vi "dump_photon_stream.vi"(5 "acq_mode":T1=2 items=["T2"=2, "T3"=3], 7 "sync":u64[](array[numeric]), 8 "error in (no error)":errorcluster, 9 "channels":u8[](array[numeric]), 10 "photon_records":u64[](array[numeric]), 11 "data_logger in":refnum<class "data_logger.lvclass">) -> (0 "error out":errorcluster, 3 "data_logger out":refnum<class "data_logger.lvclass">)   [LabVIEW 2015, in "data_logger.lvclass"]
uses:
  data_logger.lvclass
  lvoop_dll-master/picoquant_Tmodes.ctl
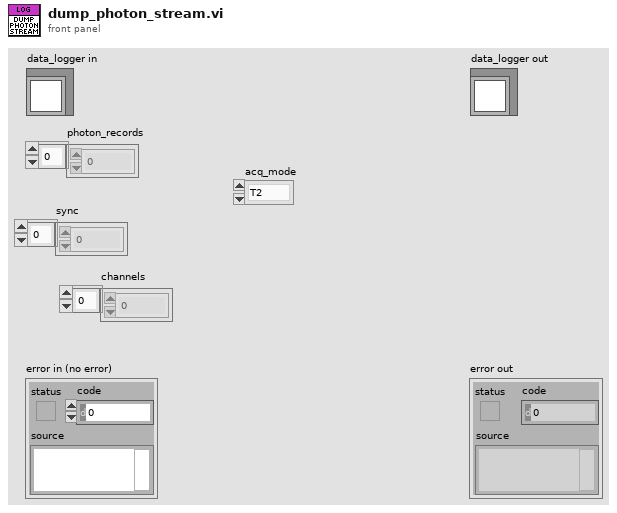
[diagram p1: front panel]
types:
  T1 = typedef "picoquant_Tmodes.ctl" = u16
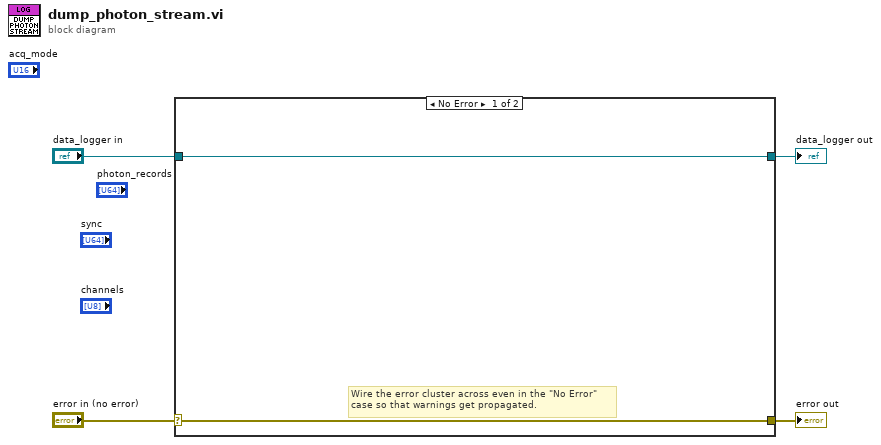
[diagram p0: block diagram]
diagram:
  n1 = case shown="No Error" "error in (no error)" {
    selector: "error in (no error)" -> [w5 w8]
    tunnel: [w5 w8] -> w3
    tunnel: [w6 w7] -> w1
    tunnel: "data_logger in" -> [w6 w7]
    frame No Error {
      # "Wire the error cluster across even in the \"No Error\"\ncase so that warnings get propagated."
    }
    frame Error {
    }
  }
  "error out" <- w3
  "data_logger out" <- w1
